vi "ConvertDataDoubleToAxisFault.vi"(8 "error in (no error)":errorcluster, 9 "Axis Fault":string(combo)="MaskValue", 10 "Double In":dbl[](array[numeric]), 11 "controller in":refnum<k24>) -> (0 "error out":errorcluster, 2 "Axis Fault Out":i32[](array[numeric]), 3 "controller out":refnum<k24>)   [LabVIEW 2021]
uses:
  C:/Program Files (x86)/Aerotech/A3200/LabVIEW/2010/Bin/Aerotech.A3200.dll
  Bin/Aerotech.A3200.dll
  C:/Program Files (x86)/Aerotech/A3200/LabVIEW/2010/Bin/Aerotech.A3200.LabVIEW.dll
  Bin/Aerotech.A3200.LabVIEW.dll
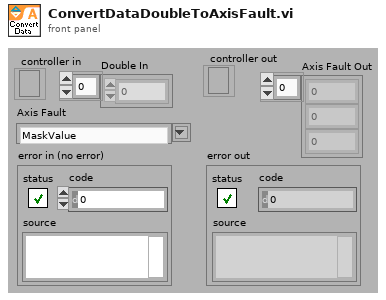
[diagram p1: front panel]
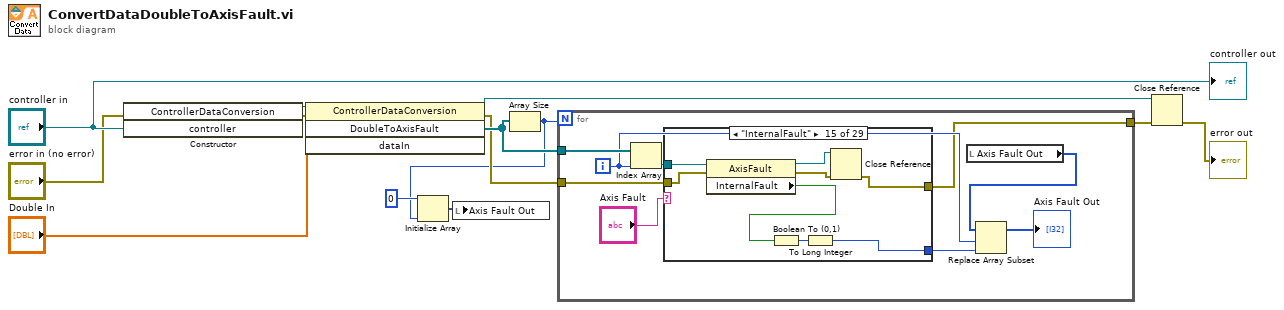
[diagram p0: block diagram]
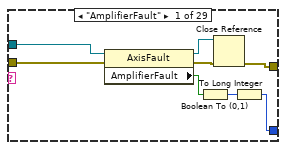
[diagram p2: hidden frame]
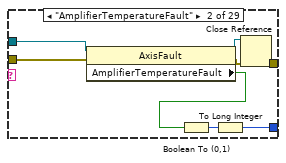
[diagram p3: hidden frame]
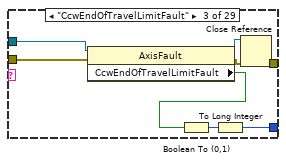
[diagram p4: hidden frame]
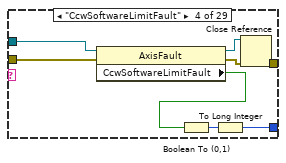
[diagram p5: hidden frame]
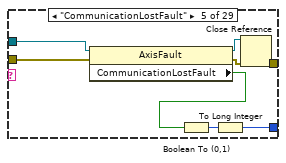
[diagram p6: hidden frame]
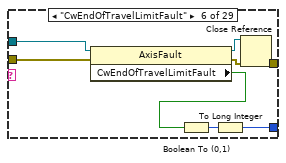
[diagram p7: hidden frame]
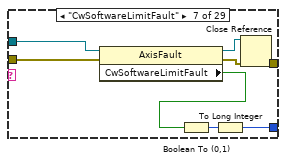
[diagram p8: hidden frame]
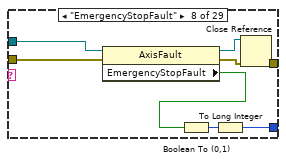
[diagram p9: hidden frame]
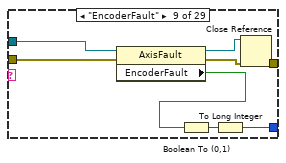
[diagram p10: hidden frame]
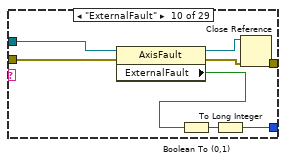
[diagram p11: hidden frame]
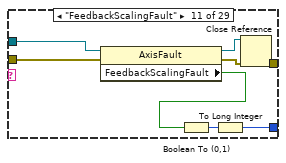
[diagram p12: hidden frame]
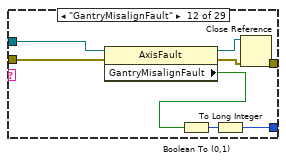
[diagram p13: hidden frame]
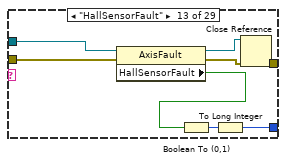
[diagram p14: hidden frame]
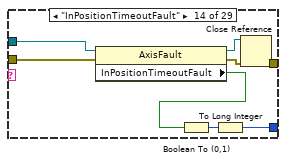
[diagram p15: hidden frame]
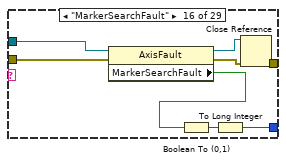
[diagram p16: hidden frame]
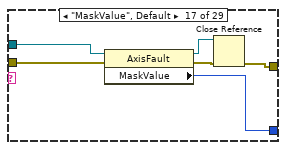
[diagram p17: hidden frame]
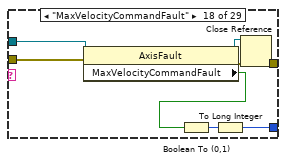
[diagram p18: hidden frame]
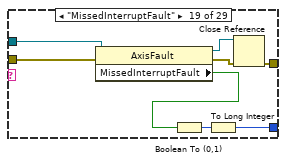
[diagram p19: hidden frame]
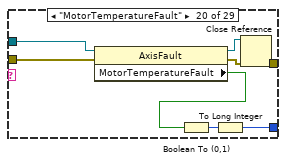
[diagram p20: hidden frame]
diagram:
  n1 = constructor class="ControllerDataConversion"(error in="error in (no error)", "controller"="controller in") -> (reference out=w13:refnum<k24>, error out=w10:errorcluster)  [unwired: 2 in, 2 out]
  n2 = invoke class="ControllerDataConversion" method="DoubleToAxisFault"(reference=w13, error in=w10, "dataIn"="Double In") -> (reference out=w8:refnum<k24>, error out=w5:errorcluster, "DoubleToAxisFault"=w6:refnum<k24>[])  [unwired: 1 in, 1 out]
  n3 = Array Size(array=w6) -> (size(s)=w2:i32)
  n4 = Initialize Array(0 ("element"), w2) -> (w1:i32[])
  n5 = local write "Axis Fault Out"(w1) -> ()
  n6 = for {
    N: w2 -> [_]
    tunnel: w6 -> [w22]
    tunnel: w5 -> [w20]
    tunnel: [w16] -> w4
    i -> [w19]
    n7 = Index Array(array=w22, index=w19) -> (element=w21:refnum<k24>)
    n8 = case shown="\"InternalFault\"" "Axis Fault" {
      tunnel: w21 -> [w30 w38 w46 w54 w62 w70 w78 w86 w94 w102 w110 w118 w126 w134 w138 w150 w156 w164 w166 w180 w188 w196 w204 w212 w220 w228 w236 w244 w252]
      tunnel: w20 -> [w27 w35 w43 w51 w59 w67 w75 w83 w91 w99 w107 w115 w123 w131 w137 w147 w153 w161 w168 w177 w185 w193 w201 w209 w217 w225 w233 w241 w249]
      tunnel: [w24 w33 w41 w49 w57 w65 w73 w81 w89 w97 w105 w113 w121 w129 w136 w145 w152 w159 w169 w175 w183 w191 w199 w207 w215 w223 w231 w239 w247] -> w17
      tunnel: [w23 w32 w40 w48 w56 w64 w72 w80 w88 w96 w104 w112 w120 w128 w135 w144 w151 w158 w167 w174 w182 w190 w198 w206 w214 w222 w230 w238 w246] -> w16
      frame "AmplifierFault" {
        n9 = property class="AxisFault"(reference=w30, error in=w27) -> (reference out=w29:refnum<k24>, error out=w28:errorcluster, "AmplifierFault"=w26:bool)
        n10 = Boolean To (0,1)(Boolean=w26) -> (0, 1=w25:i16)
        n11 = Close Reference(reference=w29, error in (no error)=w28) -> (error out=w23:errorcluster)
        n12 = To Long Integer(number=w25) -> (32bit integer=w24:i32)
      }
      frame "AmplifierTemperatureFault" {
        n13 = property class="AxisFault"(reference=w38, error in=w35) -> (reference out=w37:refnum<k24>, error out=w36:errorcluster, "AmplifierTemperatureFault"=w31:bool)
        n14 = Boolean To (0,1)(Boolean=w31) -> (0, 1=w34:i16)
        n15 = To Long Integer(number=w34) -> (32bit integer=w33:i32)
        n16 = Close Reference(reference=w37, error in (no error)=w36) -> (error out=w32:errorcluster)
      }
      frame "CcwEndOfTravelLimitFault" {
        n17 = property class="AxisFault"(reference=w46, error in=w43) -> (reference out=w45:refnum<k24>, error out=w44:errorcluster, "CcwEndOfTravelLimitFault"=w39:bool)
        n18 = Boolean To (0,1)(Boolean=w39) -> (0, 1=w42:i16)
        n19 = To Long Integer(number=w42) -> (32bit integer=w41:i32)
        n20 = Close Reference(reference=w45, error in (no error)=w44) -> (error out=w40:errorcluster)
      }
      frame "CcwSoftwareLimitFault" {
        n21 = property class="AxisFault"(reference=w54, error in=w51) -> (reference out=w53:refnum<k24>, error out=w52:errorcluster, "CcwSoftwareLimitFault"=w47:bool)
        n22 = Boolean To (0,1)(Boolean=w47) -> (0, 1=w50:i16)
        n23 = To Long Integer(number=w50) -> (32bit integer=w49:i32)
        n24 = Close Reference(reference=w53, error in (no error)=w52) -> (error out=w48:errorcluster)
      }
      frame "CommunicationLostFault" {
        n25 = property class="AxisFault"(reference=w62, error in=w59) -> (reference out=w61:refnum<k24>, error out=w60:errorcluster, "CommunicationLostFault"=w55:bool)
        n26 = Boolean To (0,1)(Boolean=w55) -> (0, 1=w58:i16)
        n27 = To Long Integer(number=w58) -> (32bit integer=w57:i32)
        n28 = Close Reference(reference=w61, error in (no error)=w60) -> (error out=w56:errorcluster)
      }
      frame "CwEndOfTravelLimitFault" {
        n29 = property class="AxisFault"(reference=w70, error in=w67) -> (reference out=w69:refnum<k24>, error out=w68:errorcluster, "CwEndOfTravelLimitFault"=w63:bool)
        n30 = Boolean To (0,1)(Boolean=w63) -> (0, 1=w66:i16)
        n31 = To Long Integer(number=w66) -> (32bit integer=w65:i32)
        n32 = Close Reference(reference=w69, error in (no error)=w68) -> (error out=w64:errorcluster)
      }
      frame "CwSoftwareLimitFault" {
        n33 = property class="AxisFault"(reference=w78, error in=w75) -> (reference out=w77:refnum<k24>, error out=w76:errorcluster, "CwSoftwareLimitFault"=w71:bool)
        n34 = Boolean To (0,1)(Boolean=w71) -> (0, 1=w74:i16)
        n35 = To Long Integer(number=w74) -> (32bit integer=w73:i32)
        n36 = Close Reference(reference=w77, error in (no error)=w76) -> (error out=w72:errorcluster)
      }
      frame "EmergencyStopFault" {
        n37 = property class="AxisFault"(reference=w86, error in=w83) -> (reference out=w85:refnum<k24>, error out=w84:errorcluster, "EmergencyStopFault"=w79:bool)
        n38 = Boolean To (0,1)(Boolean=w79) -> (0, 1=w82:i16)
        n39 = To Long Integer(number=w82) -> (32bit integer=w81:i32)
        n40 = Close Reference(reference=w85, error in (no error)=w84) -> (error out=w80:errorcluster)
      }
      frame "EncoderFault" {
        n41 = property class="AxisFault"(reference=w94, error in=w91) -> (reference out=w93:refnum<k24>, error out=w92:errorcluster, "EncoderFault"=w87:bool)
        n42 = Boolean To (0,1)(Boolean=w87) -> (0, 1=w90:i16)
        n43 = To Long Integer(number=w90) -> (32bit integer=w89:i32)
        n44 = Close Reference(reference=w93, error in (no error)=w92) -> (error out=w88:errorcluster)
      }
      frame "ExternalFault" {
        n45 = property class="AxisFault"(reference=w102, error in=w99) -> (reference out=w101:refnum<k24>, error out=w100:errorcluster, "ExternalFault"=w95:bool)
        n46 = Boolean To (0,1)(Boolean=w95) -> (0, 1=w98:i16)
        n47 = To Long Integer(number=w98) -> (32bit integer=w97:i32)
        n48 = Close Reference(reference=w101, error in (no error)=w100) -> (error out=w96:errorcluster)
      }
      frame "FeedbackScalingFault" {
        n49 = property class="AxisFault"(reference=w110, error in=w107) -> (reference out=w109:refnum<k24>, error out=w108:errorcluster, "FeedbackScalingFault"=w103:bool)
        n50 = Boolean To (0,1)(Boolean=w103) -> (0, 1=w106:i16)
        n51 = To Long Integer(number=w106) -> (32bit integer=w105:i32)
        n52 = Close Reference(reference=w109, error in (no error)=w108) -> (error out=w104:errorcluster)
      }
      frame "GantryMisalignFault" {
        n53 = property class="AxisFault"(reference=w118, error in=w115) -> (reference out=w117:refnum<k24>, error out=w116:errorcluster, "GantryMisalignFault"=w111:bool)
        n54 = Boolean To (0,1)(Boolean=w111) -> (0, 1=w114:i16)
        n55 = To Long Integer(number=w114) -> (32bit integer=w113:i32)
        n56 = Close Reference(reference=w117, error in (no error)=w116) -> (error out=w112:errorcluster)
      }
      frame "HallSensorFault" {
        n57 = property class="AxisFault"(reference=w126, error in=w123) -> (reference out=w125:refnum<k24>, error out=w124:errorcluster, "HallSensorFault"=w119:bool)
        n58 = Boolean To (0,1)(Boolean=w119) -> (0, 1=w122:i16)
        n59 = To Long Integer(number=w122) -> (32bit integer=w121:i32)
        n60 = Close Reference(reference=w125, error in (no error)=w124) -> (error out=w120:errorcluster)
      }
      frame "InPositionTimeoutFault" {
        n61 = property class="AxisFault"(reference=w134, error in=w131) -> (reference out=w133:refnum<k24>, error out=w132:errorcluster, "InPositionTimeoutFault"=w127:bool)
        n62 = Boolean To (0,1)(Boolean=w127) -> (0, 1=w130:i16)
        n63 = To Long Integer(number=w130) -> (32bit integer=w129:i32)
        n64 = Close Reference(reference=w133, error in (no error)=w132) -> (error out=w128:errorcluster)
      }
      frame "InternalFault" {
        n65 = property class="AxisFault"(reference=w138, error in=w137) -> (reference out=w142:refnum<k24>, error out=w141:errorcluster, "InternalFault"=w139:bool)
        n66 = Boolean To (0,1)(Boolean=w139) -> (0, 1=w140:i16)
        n67 = To Long Integer(number=w140) -> (32bit integer=w136:i32)
        n68 = Close Reference(reference=w142, error in (no error)=w141) -> (error out=w135:errorcluster)
      }
      frame "MarkerSearchFault" {
        n69 = property class="AxisFault"(reference=w150, error in=w147) -> (reference out=w149:refnum<k24>, error out=w148:errorcluster, "MarkerSearchFault"=w143:bool)
        n70 = Boolean To (0,1)(Boolean=w143) -> (0, 1=w146:i16)
        n71 = To Long Integer(number=w146) -> (32bit integer=w145:i32)
        n72 = Close Reference(reference=w149, error in (no error)=w148) -> (error out=w144:errorcluster)
      }
      frame "MaskValue", Default {
        n73 = property class="AxisFault"(reference=w156, error in=w153) -> (reference out=w155:refnum<k24>, error out=w154:errorcluster, "MaskValue"=w152:i32)
        n74 = Close Reference(reference=w155, error in (no error)=w154) -> (error out=w151:errorcluster)
      }
      frame "MaxVelocityCommandFault" {
        n75 = property class="AxisFault"(reference=w164, error in=w161) -> (reference out=w163:refnum<k24>, error out=w162:errorcluster, "MaxVelocityCommandFault"=w157:bool)
        n76 = Boolean To (0,1)(Boolean=w157) -> (0, 1=w160:i16)
        n77 = To Long Integer(number=w160) -> (32bit integer=w159:i32)
        n78 = Close Reference(reference=w163, error in (no error)=w162) -> (error out=w158:errorcluster)
      }
      frame "MissedInterruptFault" {
        n79 = property class="AxisFault"(reference=w166, error in=w168) -> (reference out=w165:refnum<k24>, error out=w170:errorcluster, "MissedInterruptFault"=w172:bool)
        n80 = Boolean To (0,1)(Boolean=w172) -> (0, 1=w171:i16)
        n81 = To Long Integer(number=w171) -> (32bit integer=w169:i32)
        n82 = Close Reference(reference=w165, error in (no error)=w170) -> (error out=w167:errorcluster)
      }
      frame "MotorTemperatureFault" {
        n83 = property class="AxisFault"(reference=w180, error in=w177) -> (reference out=w179:refnum<k24>, error out=w178:errorcluster, "MotorTemperatureFault"=w173:bool)
        n84 = Boolean To (0,1)(Boolean=w173) -> (0, 1=w176:i16)
        n85 = To Long Integer(number=w176) -> (32bit integer=w175:i32)
        n86 = Close Reference(reference=w179, error in (no error)=w178) -> (error out=w174:errorcluster)
      }
      frame "None" {
        n87 = property class="AxisFault"(reference=w188, error in=w185) -> (reference out=w187:refnum<k24>, error out=w186:errorcluster, "None"=w181:bool)
        n88 = Boolean To (0,1)(Boolean=w181) -> (0, 1=w184:i16)
        n89 = To Long Integer(number=w184) -> (32bit integer=w183:i32)
        n90 = Close Reference(reference=w187, error in (no error)=w186) -> (error out=w182:errorcluster)
      }
      frame "OverCurrentFault" {
        n91 = property class="AxisFault"(reference=w196, error in=w193) -> (reference out=w195:refnum<k24>, error out=w194:errorcluster, "OverCurrentFault"=w189:bool)
        n92 = Boolean To (0,1)(Boolean=w189) -> (0, 1=w192:i16)
        n93 = To Long Integer(number=w192) -> (32bit integer=w191:i32)
        n94 = Close Reference(reference=w195, error in (no error)=w194) -> (error out=w190:errorcluster)
      }
      frame "PositionErrorFault" {
        n95 = property class="AxisFault"(reference=w204, error in=w201) -> (reference out=w203:refnum<k24>, error out=w202:errorcluster, "PositionErrorFault"=w197:bool)
        n96 = Boolean To (0,1)(Boolean=w197) -> (0, 1=w200:i16)
        n97 = To Long Integer(number=w200) -> (32bit integer=w199:i32)
        n98 = Close Reference(reference=w203, error in (no error)=w202) -> (error out=w198:errorcluster)
      }
      frame "PositionFeedbackFault" {
        n99 = property class="AxisFault"(reference=w212, error in=w209) -> (reference out=w211:refnum<k24>, error out=w210:errorcluster, "PositionFeedbackFault"=w205:bool)
        n100 = Boolean To (0,1)(Boolean=w205) -> (0, 1=w208:i16)
        n101 = To Long Integer(number=w208) -> (32bit integer=w207:i32)
        n102 = Close Reference(reference=w211, error in (no error)=w210) -> (error out=w206:errorcluster)
      }
      frame "ProbeInputFault" {
        n103 = property class="AxisFault"(reference=w220, error in=w217) -> (reference out=w219:refnum<k24>, error out=w218:errorcluster, "ProbeInputFault"=w213:bool)
        n104 = Boolean To (0,1)(Boolean=w213) -> (0, 1=w216:i16)
        n105 = To Long Integer(number=w216) -> (32bit integer=w215:i32)
        n106 = Close Reference(reference=w219, error in (no error)=w218) -> (error out=w214:errorcluster)
      }
      frame "SafeZoneFault" {
        n107 = property class="AxisFault"(reference=w228, error in=w225) -> (reference out=w227:refnum<k24>, error out=w226:errorcluster, "SafeZoneFault"=w221:bool)
        n108 = Boolean To (0,1)(Boolean=w221) -> (0, 1=w224:i16)
        n109 = To Long Integer(number=w224) -> (32bit integer=w223:i32)
        n110 = Close Reference(reference=w227, error in (no error)=w226) -> (error out=w222:errorcluster)
      }
      frame "VelocityErrorFault" {
        n111 = property class="AxisFault"(reference=w236, error in=w233) -> (reference out=w235:refnum<k24>, error out=w234:errorcluster, "VelocityErrorFault"=w229:bool)
        n112 = Boolean To (0,1)(Boolean=w229) -> (0, 1=w232:i16)
        n113 = To Long Integer(number=w232) -> (32bit integer=w231:i32)
        n114 = Close Reference(reference=w235, error in (no error)=w234) -> (error out=w230:errorcluster)
      }
      frame "VelocityFeedbackFault" {
        n115 = property class="AxisFault"(reference=w244, error in=w241) -> (reference out=w243:refnum<k24>, error out=w242:errorcluster, "VelocityFeedbackFault"=w237:bool)
        n116 = Boolean To (0,1)(Boolean=w237) -> (0, 1=w240:i16)
        n117 = To Long Integer(number=w240) -> (32bit integer=w239:i32)
        n118 = Close Reference(reference=w243, error in (no error)=w242) -> (error out=w238:errorcluster)
      }
      frame "VoltageClampFault" {
        n119 = property class="AxisFault"(reference=w252, error in=w249) -> (reference out=w251:refnum<k24>, error out=w250:errorcluster, "VoltageClampFault"=w245:bool)
        n120 = Boolean To (0,1)(Boolean=w245) -> (0, 1=w248:i16)
        n121 = To Long Integer(number=w248) -> (32bit integer=w247:i32)
        n122 = Close Reference(reference=w251, error in (no error)=w250) -> (error out=w246:errorcluster)
      }
    }
    n123 = local read "Axis Fault Out"() -> (w14:i32[])
    n124 = Replace Array Subset(array=w14, new element=w17, index=w19) -> (→"Axis Fault Out":i32[])
  }
  n125 = Close Reference(reference=w8, error in (no error)=w4) -> (error out=→"error out":errorcluster)
  "controller out" <- "controller in"
